vi "Set Use Default Value.vi"(10 "error in (no error)":errorcluster, 11 "Terminal":refnum<vi>) -> (2 "error out":errorcluster)   [LabVIEW 2020, in "FlexBlocks.lvlib"]
uses:
  FlexBlocks.lvlib
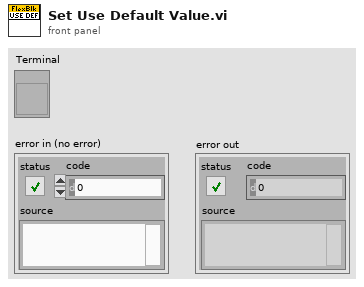
[diagram p1: front panel]
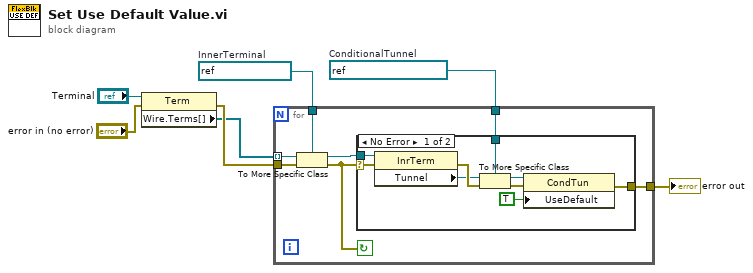
[diagram p0: block diagram]
diagram:
  w4 = refnum<vi> refnum  # ConditionalTunnel
  w5 = refnum<vi> refnum  # InnerTerminal
  n1 = property class="Term"(reference="Terminal", error in="error in (no error)") -> (error out=w7:errorcluster, "Wire.Terms[]"=w1:refnum<vi>[])  [unwired: 1 out]
  n2 = for {
    tunnel: w5 -> [w13]
    tunnel: w4 -> [w11]
    tunnel: w1 -> [w9] mode=indexing
    tunnel: w7 -> [w14]
    tunnel: [w10] -> w3
    stop <- w8 continue-if-true
    n3 = To More Specific Class(target class=w13, reference=w9, error in=w14) -> (specific class reference=w12:refnum<vi>, error out=w8:errorcluster)
    n4 = case shown="No Error" w8 {
      selector: w8 -> [w15 w24]
      tunnel: w12 -> [w22 _]
      tunnel: w11 -> [w20 _]
      tunnel: [w16 w24] -> w10
      frame No Error {
        n5 = property class="InrTerm"(reference=w22, error in=w15) -> (error out=w23:errorcluster, "Tunnel"=w21:refnum<vi>)  [unwired: 1 out]
        n6 = To More Specific Class(target class=w20, reference=w21, error in=w23) -> (specific class reference=w19:refnum<vi>, error out=w17:errorcluster)
        n7 = property class="CondTun"(reference=w19, error in=w17, "UseDefault"=TRUE ("Use Default if Unwired")) -> (error out=w16:errorcluster)  [unwired: 1 out]
      }
      frame Error {
      }
    }
  }
  "error out" <- w3
